vi "component_specification_dialog_with_user.vi"(7 "start path":path, 8 "error in (no error)":errorcluster, 11 "component specification in":T1) -> (0 "error out":errorcluster, 2 "cancelled?":bool, 3 "component specification out":T1)   [LabVIEW 2010]
uses:
  xcontrols/XUserDropdown/XUserDropdown/XUserDropdown.xctl
  xcontrols/XComponentSpecification/XComponentSpecification/XComponentSpecification.xctl
  xcontrols/XComponentSpecification/XComponentSpecification/data.ctl
  classes/ErrorController/ErrorController/class_data.vi
  classes/ErrorController/ErrorController/ErrorController.lvclass
panel:
  in  "cancelButton":bool
  in  "okButton":bool
  in  "component spec":T2(xcontrol)
  in  "user":string(xcontrol)
  # "Specify component..."
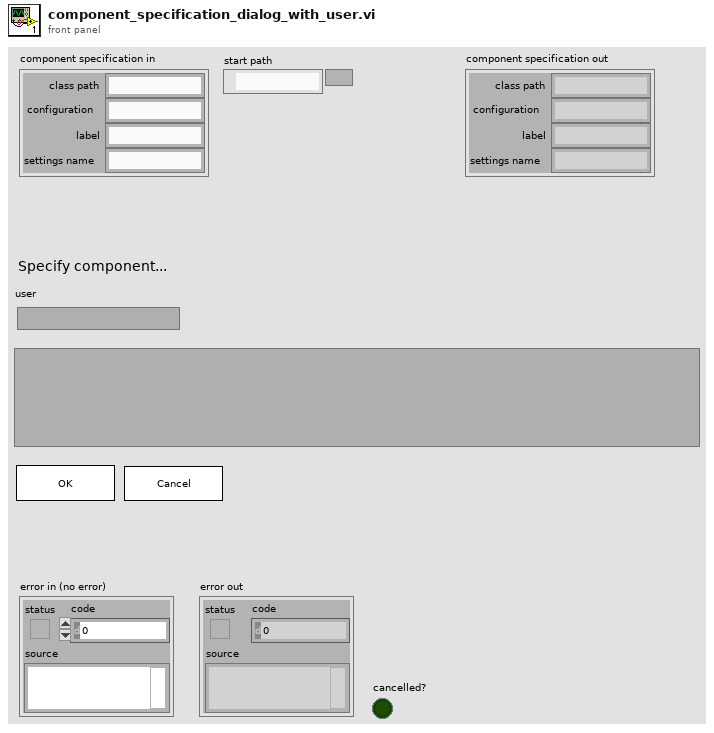
[diagram p1: front panel]
types:
  T1 = typedef "XComponentSpecification.xctl/data.ctl" = cluster{"class path":string, "configuration":string, "label":string, "settings name":string}
  T2 = cluster{"class path":string, "configuration":string, "label":string, "settings name":string}
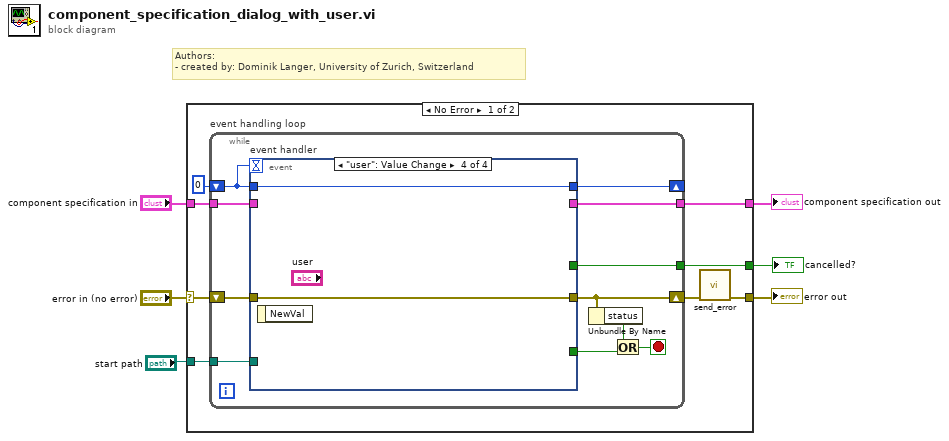
[diagram p0: block diagram]
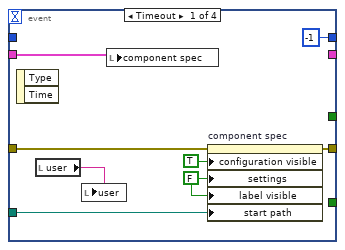
[diagram p2: hidden frame]
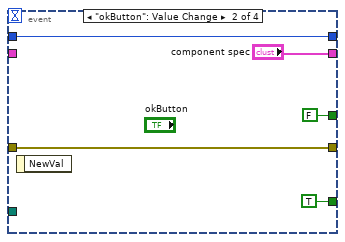
[diagram p3: hidden frame]
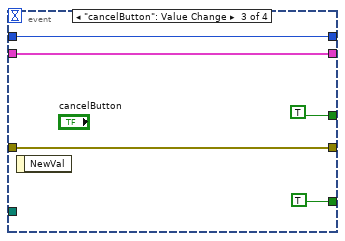
[diagram p4: hidden frame]
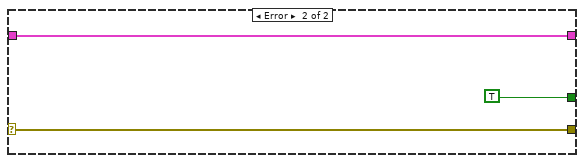
[diagram p5: hidden frame]
diagram:
  # "Authors: \n- created by: Dominik Langer, University of Zurich, Switzerland"
  n1 = case shown="No Error" "error in (no error)" {
    selector: "error in (no error)" -> [w14 w48]
    tunnel: [w7 w48] -> w5
    tunnel: [w13 TRUE] -> w4
    tunnel: "component specification in" -> [w12 w46]
    tunnel: [w11 w46] -> w2
    tunnel: "start path" -> [w9 _]
    frame No Error {
      n2 = while "event handling loop" {
        shift-right: [w18] -> w8
        shift-left: w14 -> [w25]
        tunnel: [w24] -> w13
        tunnel: w12 -> [w23]
        tunnel: [w22] -> w11
        shift-right: [w20] -> _
        shift-left: 0 -> [w21]
        tunnel: w9 -> [w19]
        stop <- w15 stop-if-true
        n3 = event "event handler" shown="[3] \"user\": Value Change" {
          selector: _ -> [_ _ _ _]
          dyn-events: _ -> [_ _ _ _]
          timeout: w21 -> [_ _ _ _]
          tunnel: w25 -> [w27 w38 w43 w45]
          tunnel: [w32 w38 w43 w45] -> w18
          tunnel: [_ FALSE TRUE _] -> w24
          tunnel: w23 -> [w29 _ w41 _]
          tunnel: [_ "component spec" w41 _] -> w22
          tunnel: [-1 w35 w40 w44] -> w20
          tunnel: w21 -> [_ w35 w40 w44]
          tunnel: [_ TRUE TRUE _] -> w16
          tunnel: w19 -> [w26 _ _ _]
          event Timeout {
            w30 = FALSE ("settings visible")
            n4 = event-data() -> ()  [unwired: 1 in, 2 out]
            n5 = local read "user"() -> (w28:string)
            n6 = local write "user"(w28) -> ()
            n7 = local write "component spec"(w29) -> ()
            n8 = property on="component spec" class="XComponentSpecification (strict"(error in=w27, "configuration visible"=TRUE, "settings"=w30, "label visible"=w30, "start path"=w26) -> (error out=w32:errorcluster)  [unwired: 1 in, 1 out]
          }
          event "okButton": Value Change {
            n9 = event-data() -> ()  [unwired: 1 in, 1 out]
          }
          event "cancelButton": Value Change {
            n10 = event-data() -> ()  [unwired: 1 in, 1 out]
          }
          event "user": Value Change {
            n11 = event-data() -> ()  [unwired: 1 in, 1 out]
          }
        }
        n12 = Unbundle By Name(w18) -> ("status"=w17:bool)
        n13 = Or(x=w17, y=w16) -> (x .or. y?=w15:bool)
      }
      n14 = call "send_error.vi"("error in (no error)"=w8) -> ("error out"=w7:errorcluster)  [unwired: 10 in]
    }
    frame Error {
    }
  }
  "error out" <- w5
  "cancelled?" <- w4
  "component specification out" <- w2
